vi "initarray.vi"(10 "size":i32, 11 "layers":i32) -> (3 "Array":i8[][][](array[numeric]))   [LabVIEW 2025]
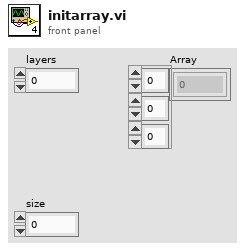
[diagram p1: front panel]
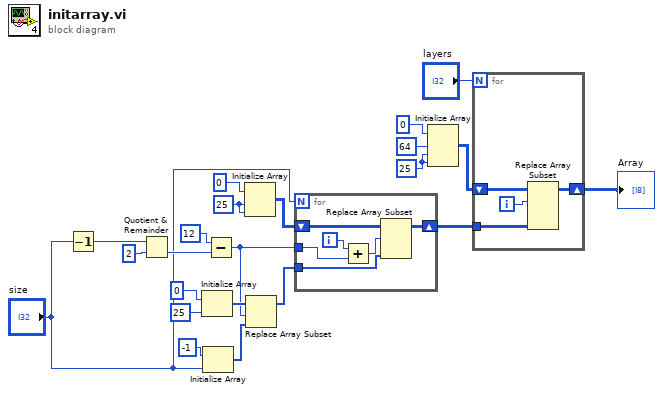
[diagram p0: block diagram]
diagram:
  w7 = 25 ("dimension size")
  w21 = 25 ("dimension size")
  n1 = Decrement(x="size") -> (x-1=w16:i32)
  n2 = Quotient & Remainder(x=w16, y=2) -> (floor(x/y)=w14:i32)  [unwired: 1 out]
  n3 = Initialize Array(i8 0 ("element"), 25 ("dimension size")) -> (w18:i8[])
  n4 = Initialize Array(i8 -1 ("element"), "size") -> (w12:i8[])
  n5 = Subtract(x=12, y=w14) -> (x-y=w10:i32)
  n6 = Initialize Array(i8 0 ("element"), w7, w7) -> (w6:i8[][])
  n7 = Replace Array Subset(array=w18, new element=w12, index=w10) -> (w11:i8[])
  n8 = for {
    N: "size" -> [_]
    tunnel: w11 -> [w28]
    tunnel: w10 -> [w24]
    shift-right: [w27] -> w4
    shift-left: w6 -> [w26]
    i -> [w25]
    n9 = Add(x=w25, y=w24) -> (x+y=w23:i32)
    n10 = Replace Array Subset(array=w26, new element=w28, index (row)=w23) -> (w27:i8[][])  [unwired: 1 in]
  }
  n11 = Initialize Array(i8 0 ("element"), 64 ("dimension size"), w21, w21) -> (w3:i8[][][])
  n12 = for {
    N: "layers" -> [_]
    tunnel: w4 -> [w32]
    shift-right: [w30] -> w1
    shift-left: w3 -> [w31]
    i -> [w29]
    n13 = Replace Array Subset(array=w31, new element=w32, index (dim 0)=w29) -> (w30:i8[][][])  [unwired: 2 in]
  }
  "Array" <- w1
